vi "X-Light V2 Send Command.vi"(0 "VISA Resource":refnum<visa-resource-name>, 7 "Command":string, 11 "Error In":errorcluster) -> (4 "VISA Resource Out":refnum<visa-resource-name>, 8 "Reply":string, 15 "Error Out":errorcluster)   [LabVIEW 2020]
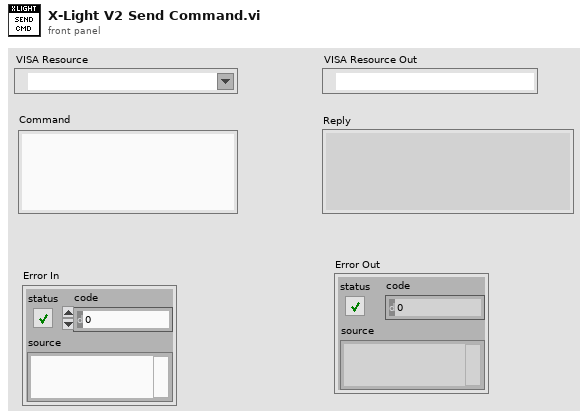
[diagram p1: front panel]
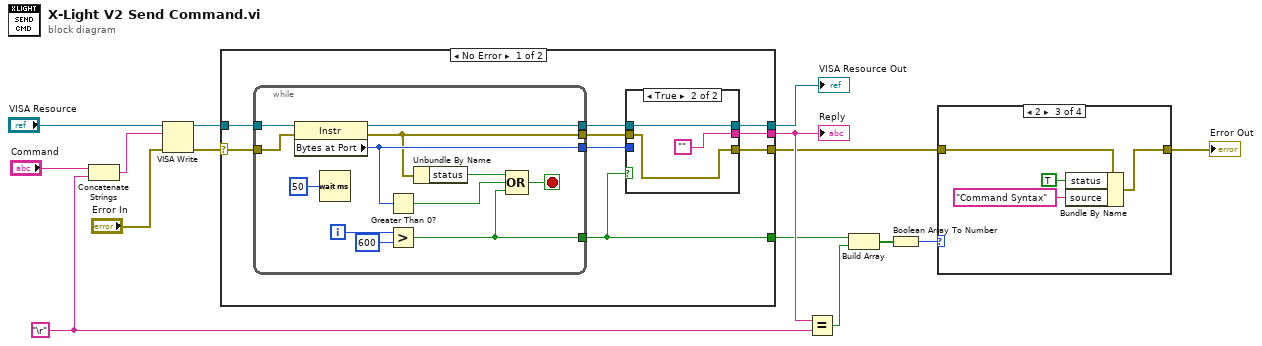
[diagram p0: block diagram]
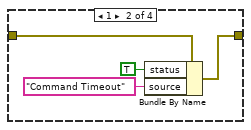
[diagram p3: hidden frame]
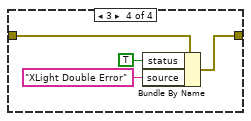
[diagram p4: hidden frame]
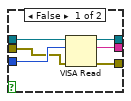
[diagram p5: hidden frame]
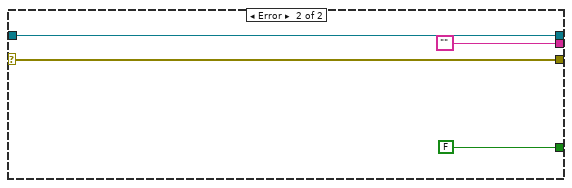
[diagram p6: hidden frame]
diagram:
  w13 = "\r"
  n1 = Concatenate Strings("Command", w13) -> (w14:string)
  n2 = VISA Write(VISA resource name="VISA Resource", write buffer=w14, error in (no error)="Error In") -> (VISA resource name out=w15:refnum<visa-resource-name>, error out=w8:errorcluster)  [unwired: 1 out]
  n3 = case shown="No Error" w8 {
    selector: w8 -> [w20 w49]
    tunnel: w15 -> [w22 w48]
    tunnel: [w19 w48] -> w10
    tunnel: [w18 w49] -> w2
    tunnel: [w17 ""] -> w7
    tunnel: [w16 FALSE] -> w6
    frame No Error {
      n4 = while {
        tunnel: [w41] -> w24
        tunnel: w20 -> [w43]
        tunnel: w22 -> [w44]
        tunnel: [w45] -> w23
        tunnel: [w38] -> w21
        tunnel: [w34] -> w16
        i -> [w40]
        stop <- w35 stop-if-true
        n5 = property class="Instr"(reference=w44, error in=w43) -> (reference out=w45:refnum<visa-resource-name>, error out=w38:errorcluster, "Bytes at Port"=w41:u32)
        n6 = Wait (ms)(milliseconds to wait=u32 50) -> ()  [unwired: 1 out]
        n7 = Greater Than 0?(x=w41) -> (x > 0?=w36:bool)
        n8 = Greater?(x=w40, y=600) -> (0:w34:bool)
        n9 = Unbundle By Name(w38) -> ("status"=w37:bool)
        n10 = Compound Arithmetic op=OR(w37, w36, w34) -> (w35:bool)
      }
      n11 = case shown="True" w16 {
        tunnel: w24 -> [w30 _]
        tunnel: w23 -> [w29 w33]
        tunnel: w21 -> [w28 w32]
        tunnel: [w27 w33] -> w19
        tunnel: [w26 w32] -> w18
        tunnel: [w25 ""] -> w17
        frame False {
          n12 = VISA Read(VISA resource name=w29, byte count=w30, error in (no error)=w28) -> (VISA resource name out=w27:refnum<visa-resource-name>, read buffer=w25:string, error out=w26:errorcluster)  [unwired: 1 out]
        }
        frame True {
        }
      }
    }
    frame Error {
    }
  }
  "Reply" <- w7
  "VISA Resource Out" <- w10
  n13 = Equal?(x=w7, y=w13) -> (x = y?=w5:bool)
  n14 = Build Array(w6, w5) -> (w4:bool[])
  n15 = Boolean Array To Number(Boolean array=w4) -> (number=w3:u32)
  n16 = case shown="2" w3 {
    tunnel: w2 -> [w50 w54 w56 w60]
    tunnel: [w50 w51 w55 w59] -> w1
    frame 0, Default {
    }
    frame 1 {
      n17 = Bundle By Name(cluster=w54, "status"=TRUE, "source"="Command Timeout") -> (w51:errorcluster)
    }
    frame 2 {
      n18 = Bundle By Name(cluster=w56, "status"=TRUE, "source"="Command Syntax") -> (w55:errorcluster)
    }
    frame 3 {
      n19 = Bundle By Name(cluster=w60, "status"=TRUE, "source"="XLight Double Error") -> (w59:errorcluster)
    }
  }
  "Error Out" <- w1
